vi "Test settings fgv.vi"(7 "Set?":bool, 8 "error in (no error)":errorcluster, 10 "Settings selected?":bool, 11 "Test settings":T1={"Speed (mm/s)"=0.0001, "Position limit"=FALSE, "Position limit (mm)"=0.0001, "Load limit"=FALSE, "Load limit (N)"=0.0001, "No. of repeats"=0, "Test identifier"="", "Time wait"=FALSE, "Wait time (s)"=0.0, "Trigger wait"=FALSE, "Send trigger"=FALSE, "Test notes"="", "Snap intervals"=FALSE, "Time interval (s)"=0.5} {"Time interval (s)" min=0.5; "No. of repeats" min=1 max=20 step=1; "Load limit (N)" min=0.0001 max=20.0 step=0.0001; "Position limit (mm)" min=0.0001 max=20.0 step=0.0001; "Speed (mm/s)" min=0.0001 max=20.0 step=0.0001}) -> (0 "error out":errorcluster, 2 "Settings selected?  out":bool, 3 "Test settings out":T1={"Speed (mm/s)"=0.0001, "Position limit"=FALSE, "Position limit (mm)"=0.0001, "Load limit"=FALSE, "Load limit (N)"=0.0001, "No. of repeats"=0, "Test identifier"="", "Time wait"=FALSE, "Wait time (s)"=0.0, "Trigger wait"=FALSE, "Send trigger"=FALSE, "Test notes"="", "Snap intervals"=FALSE, "Time interval (s)"=0.5} {"Time interval (s)" min=0.5; "No. of repeats" min=1 max=20 step=1; "Load limit (N)" min=0.0001 max=20.0 step=0.0001; "Position limit (mm)" min=0.0001 max=20.0 step=0.0001; "Speed (mm/s)" min=0.0001 max=20.0 step=0.0001})   [LabVIEW 2016]
uses:
  Controls/Test settings.ctl
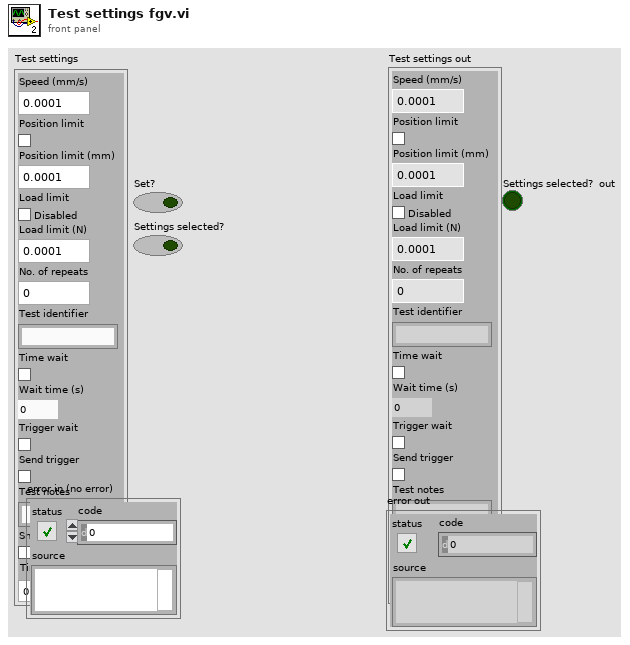
[diagram p1: front panel]
types:
  T1 = typedef "Test settings.ctl" = cluster{"Speed (mm/s)":dbl, "Position limit":bool, "Position limit (mm)":dbl, "Load limit":bool, "Load limit (N)":dbl, "No. of repeats":u16, "Test identifier":string, "Time wait":bool, "Wait time (s)":dbl, "Trigger wait":bool, "Send trigger":bool, "Test notes":string, "Snap intervals":bool, "Time interval (s)":dbl}
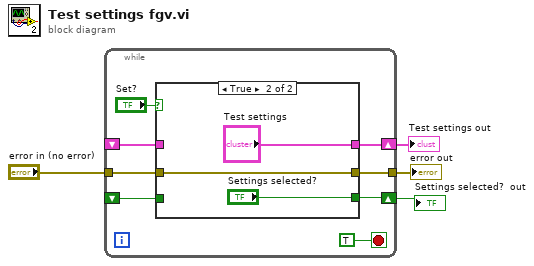
[diagram p0: block diagram]
diagram:
  n1 = while {
    shift-right: [w10] -> w4
    shift-left: _ -> [w9]
    tunnel: "error in (no error)" -> [w8]
    tunnel: [w7] -> w2
    shift-right: [w5] -> w1
    shift-left: _ -> [w6]
    stop <- TRUE stop-if-true
    n2 = case shown="True" "Set?" {
      tunnel: [w15 "Test settings"] -> w10
      tunnel: w9 -> [w15 _]
      tunnel: w8 -> [w14 w17]
      tunnel: [w14 w17] -> w7
      tunnel: w6 -> [w13 _]
      tunnel: [w13 "Settings selected?"] -> w5
      frame False {
      }
      frame True {
      }
    }
  }
  "Test settings out" <- w4
  "error out" <- w2
  "Settings selected?  out" <- w1
